vi "txt2Json.vi"(5 "uploadPath":path, 7 "failpath":path=path "d:/xmlconvert/success", 8 "错误输入":errorcluster caption="error In", 9 "successpath":path=path "d:/xmlconvert/success", 10 "statusRef":refnum<vi>, 11 "TGA/DSC new data":T2) -> (0 "错误输出":errorcluster caption="error Out")   [LabVIEW 2011]
uses:
  dataType/TGA_DSC new data record.ctl
  dataType/TGA_DSC.ctl
panel:
  in  "DBSet":T1={"Server"="172.20.23.107", "DB"="MESDATACenter", "PSW"="data'songyy", "User"="sa"}
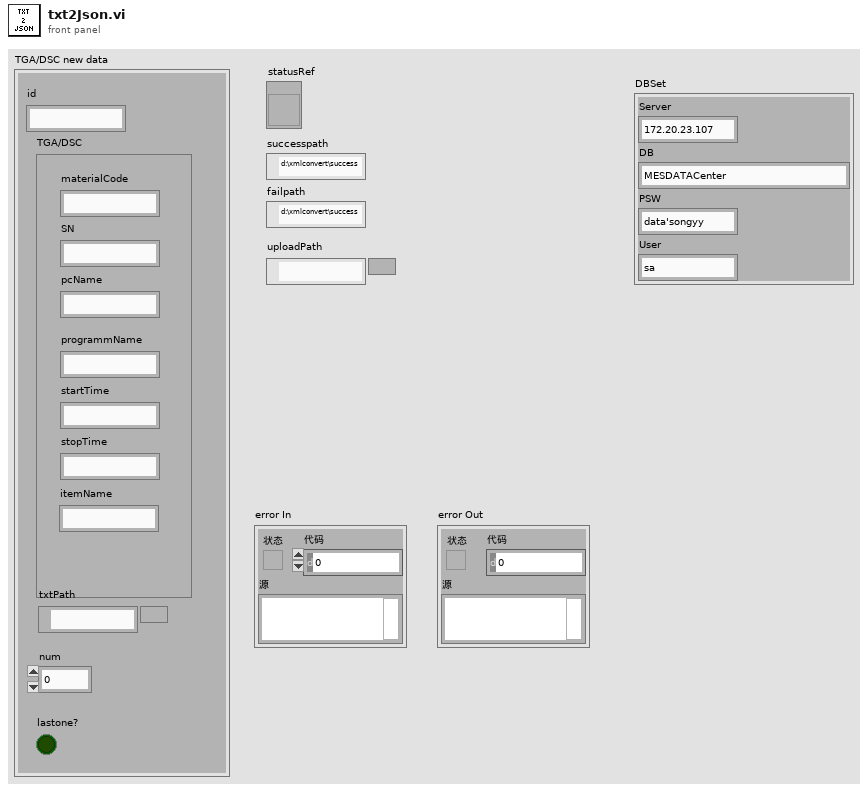
[diagram p1: front panel]
types:
  T1 = cluster{"Server":string, "DB":string, "PSW":string, "User":string}
  T2 = typedef "TGA_DSC new data record.ctl" = cluster{"id":string, "TGA/DSC":T3, "txtPath":path, "num":dbl, "lastone?":bool}
  T3 = typedef "TGA_DSC.ctl" = cluster{"materialCode":string, "SN":string, "pcName":string, "programmName":string, "startTime":string, "stopTime":string, "itemName":string}
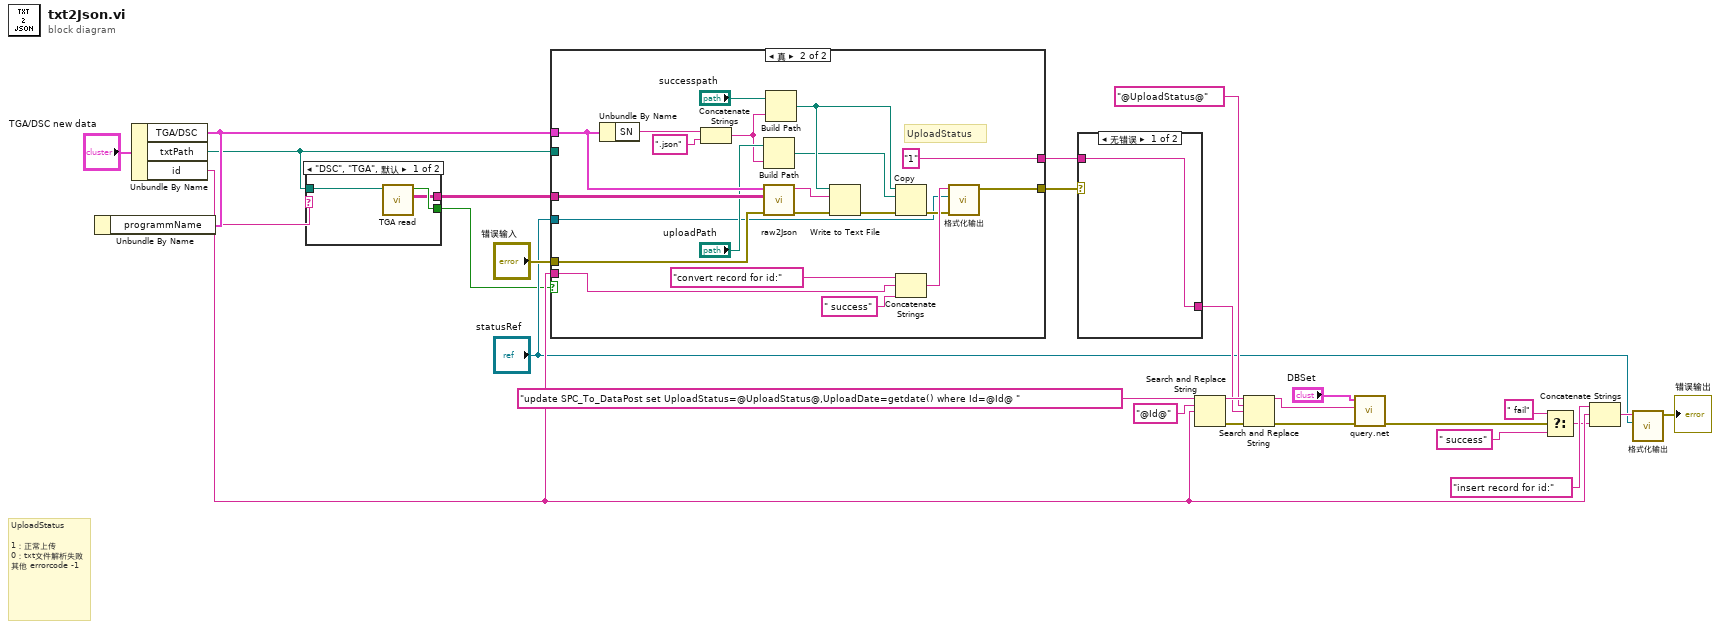
[diagram p0: block diagram]
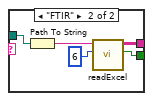
[diagram p2: hidden frame]
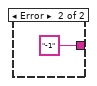
[diagram p3: hidden frame]
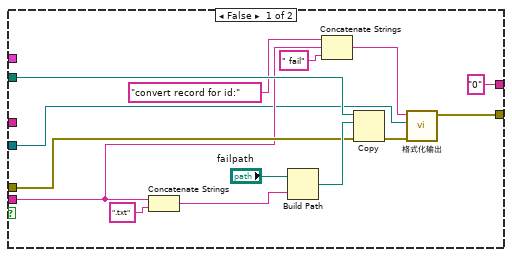
[diagram p4: hidden frame]
diagram:
  # "UploadStatus\n\n1：正常上传\n0：txt文件解析失败\n其他 errorcode -1"
  n1 = Unbundle By Name("TGA/DSC new data") -> ("TGA/DSC"=w5:T3, "txtPath"=w4:path, "id"=w14:string)
  n2 = Unbundle By Name(w5) -> ("programmName"=w1:string)
  n3 = case shown="\"DSC\", \"TGA\", 默认" w1 {
    tunnel: w4 -> [w30 w32]
    tunnel: [w29 w33] -> w3
    tunnel: [w28 w34] -> w2
    frame "DSC", "TGA", Default {
      n4 = call "TGA read.vi"("file path (dialog if empty)"=w30) -> ("rawData"=w28:string[][], "dataCheckOK"=w29:bool)  [unwired: 9 in]
    }
    frame "FTIR" {
      n5 = Path To String(path=w32) -> (string=w31:string)
      n6 = call "readExcel.vi"("StartRow"=6, "XlsPath"=w31) -> ("dataCheckOK"=w33:bool, "getXYValue_string"=w34:string[][])  [unwired: 7 in, 1 out]
    }
  }
  n7 = case shown="真" w3 {
    tunnel: w5 -> [_ w69]
    tunnel: w2 -> [_ w70]
    tunnel: w4 -> [w46 _]
    tunnel: w14 -> [w40 w53]
    tunnel: [w37 w51] -> w25
    tunnel: "错误输入" -> [w44 w59]
    tunnel: ["0" "1"] -> w24
    tunnel: "statusRef" -> [w36 w50]
    frame False {
      n8 = Concatenate Strings(w40, ".txt" ("字符串")) -> (w47:string)
      n9 = Build Path(base path="failpath", name or relative path=w47) -> (appended path=w45:path)
      n10 = Concatenate Strings("convert record for id:", w40, " fail" ("字符串")) -> (w41:string)
      n11 = Copy(8:w44, 10:w45, 11:w46) -> (0:w38:errorcluster)  [unwired: 2 in, 2 out]
      n12 = call "格式化输出.vi"("错误输入（无错误）"=w38, "字符串引用"=w36, "字符串"=w41) -> ("错误输出"=w37:errorcluster)  [unwired: 8 in]
    }
    frame True {
      # "UploadStatus"
      n13 = Unbundle By Name(w69) -> ("SN"=w68:string)
      n14 = Concatenate Strings(w68, ".json" ("字符串")) -> (w61:string)
      n15 = Build Path(base path="uploadPath", name or relative path=w61) -> (appended path=w60:path)
      n16 = call "raw2Json.vi"("error in"=w59, "rawData"=w70, "TGA/DSC"=w69) -> ("error in 2"=w58:errorcluster, "fullJson"=w66:string)  [unwired: 7 in]
      n17 = Build Path(base path="successpath", name or relative path=w61) -> (appended path=w64:path)
      n18 = Write to Text File(file (use dialog)=w64, text=w66, error in=w58) -> (error out=w63:errorcluster)  [unwired: 1 in, 2 out]
      n19 = Copy(8:w63, 10:w60, 11:w64) -> (0:w52:errorcluster)  [unwired: 2 in, 2 out]
      n20 = Concatenate Strings("convert record for id:", w53, " success" ("字符串")) -> (w55:string)
      n21 = call "格式化输出.vi"("错误输入（无错误）"=w52, "字符串引用"=w50, "字符串"=w55) -> ("错误输出"=w51:errorcluster)  [unwired: 8 in]
    }
  }
  n22 = case shown="无错误" w25 {
    tunnel: w24 -> [w71 _]
    tunnel: [w71 "-1"] -> w19
    frame No Error {
    }
    frame Error {
    }
  }
  n23 = Search and Replace String(input string="update SPC_To_DataPost set UploadStatus=@UploadStatus@,UploadDate=getdate() where Id=@Id@ " ("Sql"), search string="@Id@" ("搜索字符串"), replace string=w14) -> (result string=w21:string, error out=w18:errorcluster)  [unwired: 5 in, 2 out]
  n24 = Search and Replace String(input string=w21, search string="@UploadStatus@" ("替换字符串(\"\")"), replace string=w19, error in=w18) -> (result string=w16:string, error out=w17:errorcluster)  [unwired: 4 in, 2 out]
  n25 = call "query.net.vi"("错误输入（无错误）"=w17, "Sql"=w16, "DBSet"="DBSet") -> ("错误输出"=w13:errorcluster)  [unwired: 7 in, 1 out]
  n26 = Select(t=" fail", s=w13, f=" success") -> (s? t:f=w10:string)
  n27 = Concatenate Strings("insert record for id:", w14, w10) -> (w9:string)
  n28 = call "格式化输出.vi"("字符串引用"="statusRef", "字符串"=w9) -> ("错误输出"=→"错误输出":errorcluster)  [unwired: 9 in]
